vi "EDS test 01_with motor and Firebase with sensors.vi"() -> ()   [LabVIEW 2020]
uses:
  <vilib>/DAQmx/read.llb/DAQmx Read (Digital Bool 1Line 1Point).vi
  <vilib>/DAQmx/read.llb/DAQmx Read (Analog DBL 1Chan 1Samp).vi
  <vilib>/DAQmx/write.llb/DAQmx Write (Digital Bool 1Line 1Point).vi
  <vilib>/Instr/_visa.llb/VISA Configure Serial Port (Instr).vi
  <vilib>/DAQmx/create/channels.llb/DAQmx Create Channel (DI-Digital Input).vi
  <vilib>/DAQmx/create/channels.llb/DAQmx Create Channel (AI-Voltage-Basic).vi
  <vilib>/DAQmx/configure/timing.llb/DAQmx Timing (Sample Clock).vi
  <vilib>/DAQmx/create/channels.llb/DAQmx Create Channel (DO-Digital Output).vi
  <vilib>/DAQmx/miscellaneous.llb/DAQmx Fill In Error Info.vi
  <vilib>/httpClient/PUTBuffer.vi
  <vilib>/httpClient/LabVIEWHTTPClient.lvlib
panel:
  out "Train Speed":string
  out "Trolley Speed":string
  out "Trolley Distance":dbl
  out "Elephant Distance":dbl
  out "IR and Force Sensor":bool
  out "Force Sensor":dbl(graph)
  out "error out":errorcluster
  out "Concatenated String":string
  out "read buffer":string
  in  "stop":bool
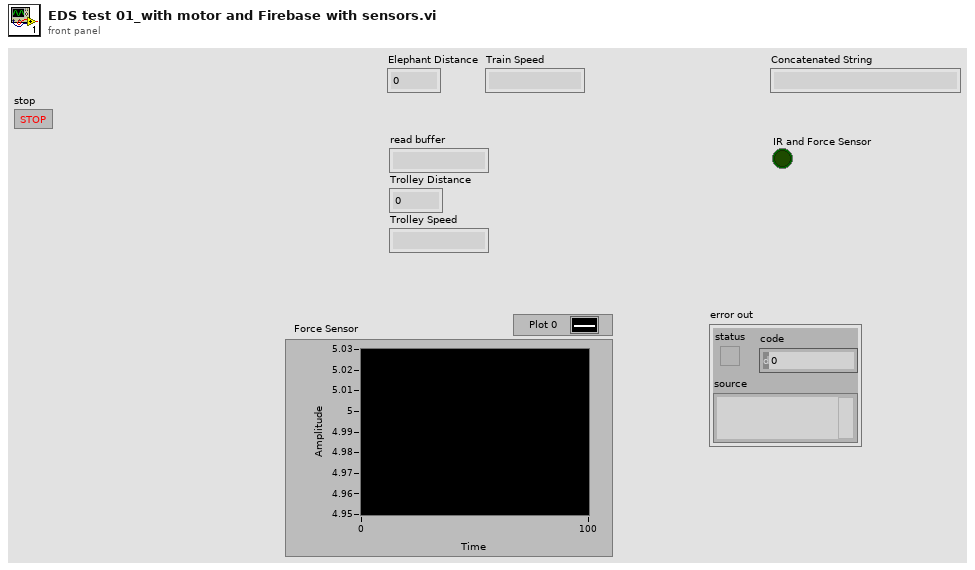
[diagram p1: front panel]
types:
  T1 = typedef "LabVIEWHTTPClient.lvlib/ClientHandle.ctl" = refnum<k1>
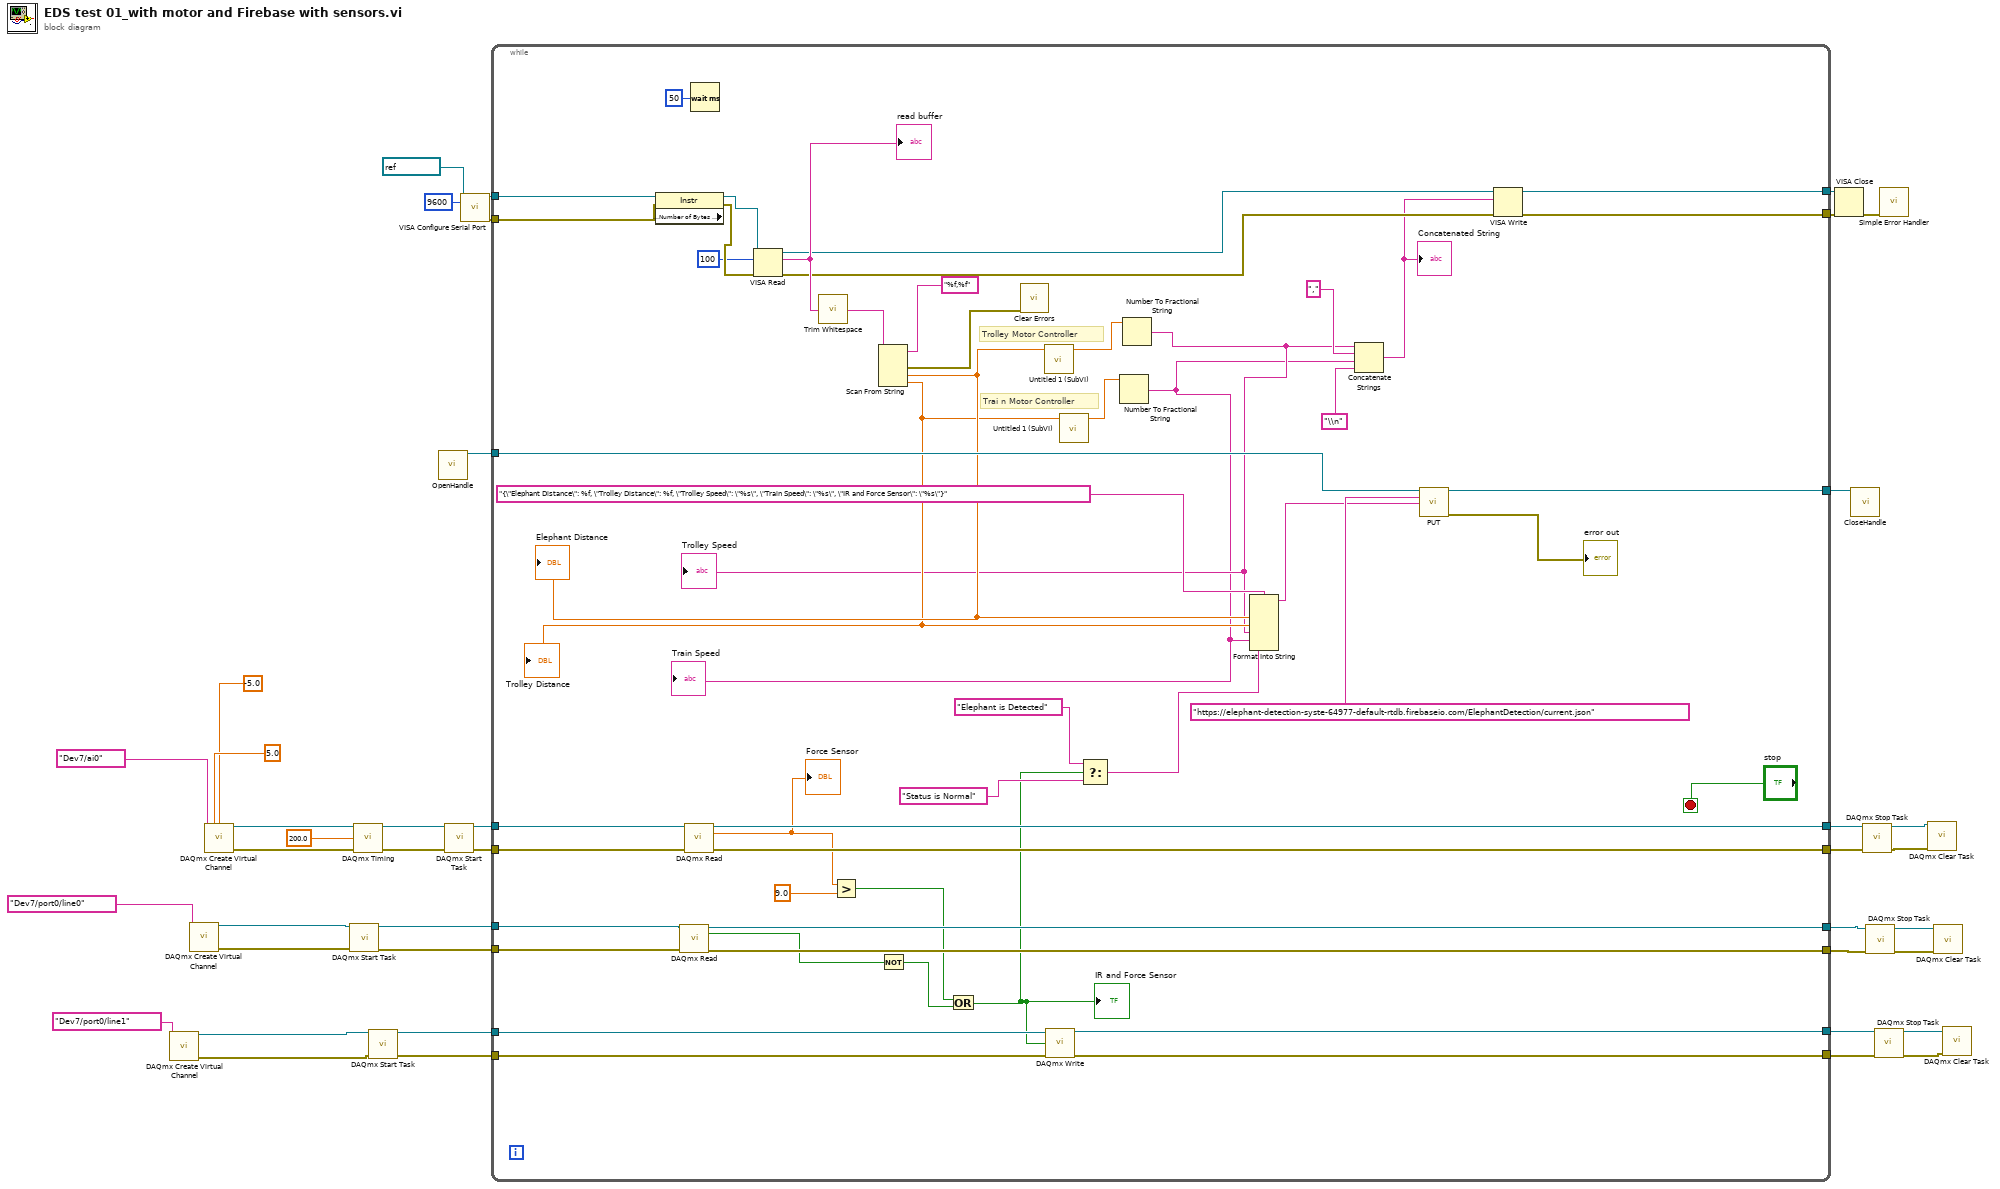
[diagram p0: block diagram]
diagram:
  n1 = call-poly <vilib>:"DAQmx Create Virtual Channel.vi"("lines"=tag "Dev7/port0/line1") -> ("task out"=w9:refnum<k21>, "error out"=w7:errorcluster)  [unwired: 13 in]
  n2 = call-poly <vilib>:"DAQmx Create Virtual Channel.vi"("lines"=tag "Dev7/port0/line0") -> ("task out"=w17:refnum<k21>, "error out"=w16:errorcluster)  [unwired: 13 in]
  n3 = call-poly <vilib>:"DAQmx Create Virtual Channel.vi"("maximum value"=5.0, "minimum value"=-5.0, "physical channels"=tag "Dev7/ai0") -> ("task out"=w32:refnum<k21>, "error out"=w23:errorcluster)  [unwired: 11 in]
  n4 = call <vilib>:"DAQmx Start Task.vi"("task/channels in"=w17, "error in"=w16) -> ("task out"=w15:refnum<k21>, "error out"=w14:errorcluster)  [unwired: 12 in]
  n5 = call-poly <vilib>:"DAQmx Timing.vi"("task/channels in"=w32, "rate"=200.0, "error in"=w23) -> ("task out"=w31:refnum<k21>, "error out"=w24:errorcluster)  [unwired: 11 in]
  n6 = call <vilib>:"DAQmx Start Task.vi"("task/channels in"=w9, "error in"=w7) -> ("task out"=w8:refnum<k21>, "error out"=w6:errorcluster)  [unwired: 12 in]
  n7 = call <vilib>:"OpenHandle.vi"() -> ("client handle out"=w34:T1)  [unwired: 14 in, 1 out]
  n8 = call <vilib>:"DAQmx Start Task.vi"("task/channels in"=w31, "error in"=w24) -> ("task out"=w30:refnum<k21>, "error out"=w25:errorcluster)  [unwired: 12 in]
  n9 = call-poly "VISA Configure Serial Port"("VISA resource name"=refnum<visa-resource-name> "COM3", "baud rate (9600)"=u32 9600) -> ("VISA resource name out"=w39:refnum<visa-resource-name>, "error out"=w38:errorcluster)  [unwired: 12 in]
  n10 = while {
    tunnel: w39 -> [w92]
    tunnel: w38 -> [w91]
    tunnel: [w77] -> w36
    tunnel: [w76] -> w35
    tunnel: w34 -> [w65]
    tunnel: [w64] -> w33
    tunnel: w30 -> [w59]
    tunnel: [w58] -> w29
    tunnel: [w57] -> w26
    tunnel: w25 -> [w56]
    tunnel: w15 -> [w54]
    tunnel: w14 -> [w53]
    tunnel: [w52] -> w13
    tunnel: [w51] -> w10
    tunnel: w8 -> [w50]
    tunnel: w6 -> [w49]
    tunnel: [w48] -> w5
    tunnel: [w47] -> w4
    stop <- "stop" stop-if-true
    # "Trai n Motor Controller"
    # "Trolley Motor Controller"
    n11 = property class="Instr" props=["Serial Settings:Number of Bytes at Serial Port"](reference=w92, error in=w91) -> (reference out=w87:refnum<visa-resource-name>, error out=w88:errorcluster)  [unwired: 1 out]
    n12 = call-poly <vilib>:"DAQmx Read.vi"("task/channels in"=w54, "error in"=w53) -> ("task out"=w52:refnum<k21>, "data"=w43:bool, "error out"=w51:errorcluster)  [unwired: 11 in]
    n13 = call-poly <vilib>:"DAQmx Read.vi"("task/channels in"=w59, "error in"=w56) -> ("task out"=w58:refnum<k21>, "data"=w45:dbl, "error out"=w57:errorcluster)  [unwired: 11 in]
    "Force Sensor" <- w45
    n14 = Wait (ms)(milliseconds to wait=u32 50) -> ()  [unwired: 1 out]
    n15 = VISA Read(VISA resource name=w87, byte count=u32 100, error in (no error)=w88) -> (VISA resource name out=w79:refnum<visa-resource-name>, read buffer=w86:string, error out=w78:errorcluster)  [unwired: 1 out]
    "read buffer" <- w86
    n16 = call <vilib>:"Trim Whitespace.vi"("string"=w86) -> ("trimmed string"=w85:string)  [unwired: 1 in]
    n17 = Greater?(x=w45, y=9.0) -> (0:w46:bool)
    n18 = Scan From String "Scan From String"(format string="%f,%f", input string=w85) -> (error out=w83:errorcluster, output 1=w63:dbl, output 2=w62:dbl)  [unwired: 4 in, 2 out]
    "Elephant Distance" <- w63
    "Trolley Distance" <- w62
    n19 = Not(x=w43) -> (.not. x?=w42:bool)
    n20 = Or(x=w46, y=w42) -> (x .or. y?=w44:bool)
    "IR and Force Sensor" <- w44
    n21 = call <vilib>:"Clear Errors.vi"("error in (no error)"=w83) -> ()  [unwired: 5 in, 2 out]
    n22 = call "Untitled 1 (SubVI).vi"("Ultrasonic 01"=w63) -> ("Numeric"=w81:dbl)  [unwired: 10 in]
    n23 = call-poly <vilib>:"DAQmx Write.vi"("task/channels in"=w50, "data"=w44, "error in"=w49) -> ("task out"=w48:refnum<k21>, "error out"=w47:errorcluster)  [unwired: 10 in, 1 out]
    n24 = call "Untitled 1 (SubVI).vi"("Ultrasonic 01"=w62) -> ("Numeric"=w80:dbl)  [unwired: 10 in]
    n25 = Select(t="Elephant is Detected" ("format string"), s=w44, f="Status is Normal" ("format string")) -> (s? t:f=w70:string)
    n26 = Number To Fractional String(number=w80) -> (F-format string=w60:string)  [unwired: 3 in]
    "Train Speed" <- w60
    n27 = Number To Fractional String(number=w81) -> (F-format string=w61:string)  [unwired: 3 in]
    "Trolley Speed" <- w61
    n28 = Format Into String(format string="{\"Elephant Distance\": %f, \"Trolley Distance\": %f, \"Trolley Speed\": \"%s\", \"Train Speed\": \"%s\", \"IR and Force Sensor\": \"%s\"}", w63, w62, w61, w60, w70) -> (resulting string=w67:string)  [unwired: 2 in, 1 out]
    n29 = Concatenate Strings "Concatenate Strings"(w61, ",", w60, "\\n") -> (w75:string)
    "Concatenated String" <- w75
    n30 = call-poly <vilib>:"PUT.vi"("client handle"=w65, "url"="https://elephant-detection-syste-64977-default-rtdb.firebaseio.com/ElephantDetection/current.json", "buffer"=w67) -> ("client handle out"=w64:T1, "error out"=→"error out":errorcluster)  [unwired: 9 in, 2 out]
    n31 = VISA Write(VISA resource name=w79, write buffer=w75, error in (no error)=w78) -> (VISA resource name out=w77:refnum<visa-resource-name>, error out=w76:errorcluster)  [unwired: 1 out]
  }
  n32 = VISA Close(VISA resource name=w36, error in (no error)=w35) -> (error out=w37:errorcluster)
  n33 = call <vilib>:"CloseHandle.vi"("client handle"=w33) -> ()  [unwired: 14 in, 1 out]
  n34 = call <vilib>:"DAQmx Stop Task.vi"("task/channels in"=w29, "error in"=w26) -> ("task out"=w28:refnum<k21>, "error out"=w27:errorcluster)  [unwired: 12 in]
  n35 = call <vilib>:"DAQmx Stop Task.vi"("task/channels in"=w13, "error in"=w10) -> ("task out"=w12:refnum<k21>, "error out"=w11:errorcluster)  [unwired: 12 in]
  n36 = call <vilib>:"DAQmx Stop Task.vi"("task/channels in"=w5, "error in"=w4) -> ("task out"=w3:refnum<k21>, "error out"=w2:errorcluster)  [unwired: 12 in]
  n37 = call <vilib>:"Simple Error Handler.vi"("error in (no error)"=w37) -> ()  [unwired: 4 in, 5 out]
  n38 = call <vilib>:"DAQmx Clear Task.vi"("task in"=w28, "error in"=w27) -> ()  [unwired: 13 in, 1 out]
  n39 = call <vilib>:"DAQmx Clear Task.vi"("task in"=w12, "error in"=w11) -> ()  [unwired: 13 in, 1 out]
  n40 = call <vilib>:"DAQmx Clear Task.vi"("task in"=w3, "error in"=w2) -> ()  [unwired: 13 in, 1 out]
